vi "DashboardGlobals.vi"() -> ()   [LabVIEW 2019]
panel:
  out "ValuesGotOverwritten":bool
  in  "CalibrationPath":string="C:\\Users\\ASUS\\Desktop\\Simulation\\"
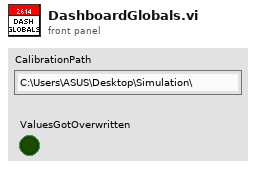
[diagram p1: front panel]
diagram:
